vi "niWLAN - 80211abgnIQMeasurementsReadWrite.vi"(0 "niwlan analysis session":T3, 1 "file path (dialog if empty)":path, 2 "Measurement Type":T1(ring), 3 "PL":dbl, 7 "TV Parameters(DataType)":T2 {"Tx_Chan" format="%.0x"; "Standard" items=["80211A/G/J/P OFDM", "80211B/G DSSS", "80211G DSSSOFDM", "80211N MIMOOFDM", "80211AC MIMOOFDM"]; "OFDM Data Rate (Mbps)" items=["6", "9", "12", "18", "24", "36", "48", "54"]; "80211n PLCP Frame Format" items=["Mixed Format", "Greenfield Format"]; "FEC Coding Type" items=["BCC", "LDPC"]; "DSSS Data Rate (Mbps)" items=["1", "2", "5.5 CCK", "5.5 PBCC", "11 CCK", "11 PBCC", "22", "33"]}, 11 "error out":errorcluster, 12 "Measurement Time":dbl[](array[numeric]), 13 "First Row":bool=TRUE) -> (4 "niWLAN session":T3, 15 "error out":errorcluster)   [LabVIEW 2011]
uses:
  <vilib>/RF Toolkits/WLAN/analysis/controls/wlanv1 Analysis Refnum.ctl
  TV/RW/Includes/WLAN - TV - RW - INC - TV_DataType_Cluster.ctl
  <vilib>/Utility/file.llb/Write To Spreadsheet File (string).vi
  Program Files/National Instruments/LabVIEW 2011/resource/objmgr/niWLANAnalysis.rc
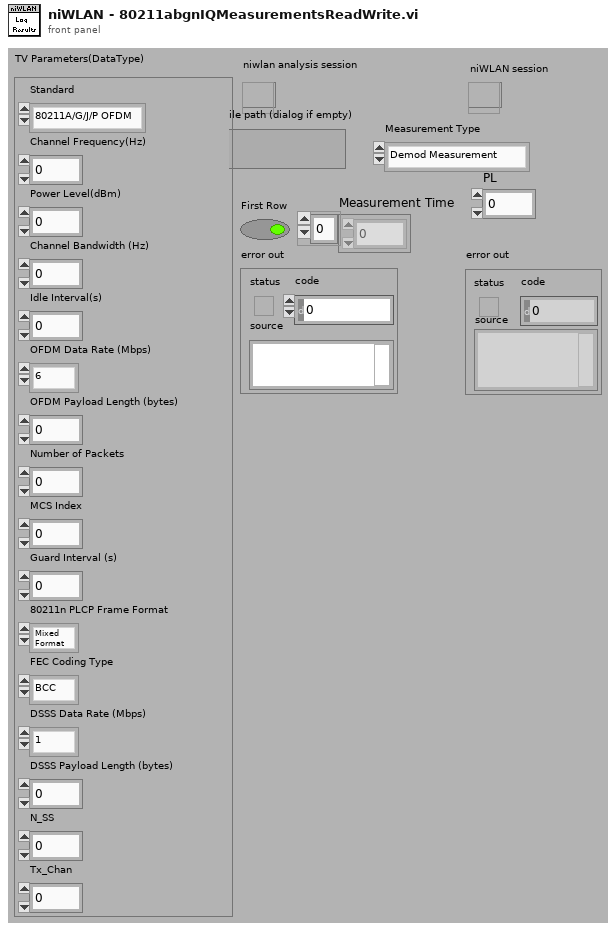
[diagram p1: front panel]
types:
  T1 = enum16{"Demod Measurement", "Spectrum Measurement"}
  T2 = typedef "WLAN - TV - RW - INC - TV_DataType_Cluster.ctl" = cluster{"Standard":i32, "Channel Frequency(Hz)":dbl, "Power Level(dBm)":dbl, "Channel Bandwidth (Hz)":dbl, "Idle Interval(s)":dbl, "OFDM Data Rate (Mbps)":i32, "OFDM Payload Length (bytes)":i32, "Number of Packets":i32, "MCS Index":i32, "Guard Interval (s)":dbl, "80211n PLCP Frame Format":i32, "FEC Coding Type":i32, "DSSS Data Rate (Mbps)":i32, "DSSS Payload Length (bytes)":i32, "N_SS":i32, "Tx_Chan":u32}
  T3 = typedef "wlanv1 Analysis Refnum.ctl" = refnum<k20>
  T4 = cluster{"subcarrier indices":i32[], "relative power (dB)":dbl[]}
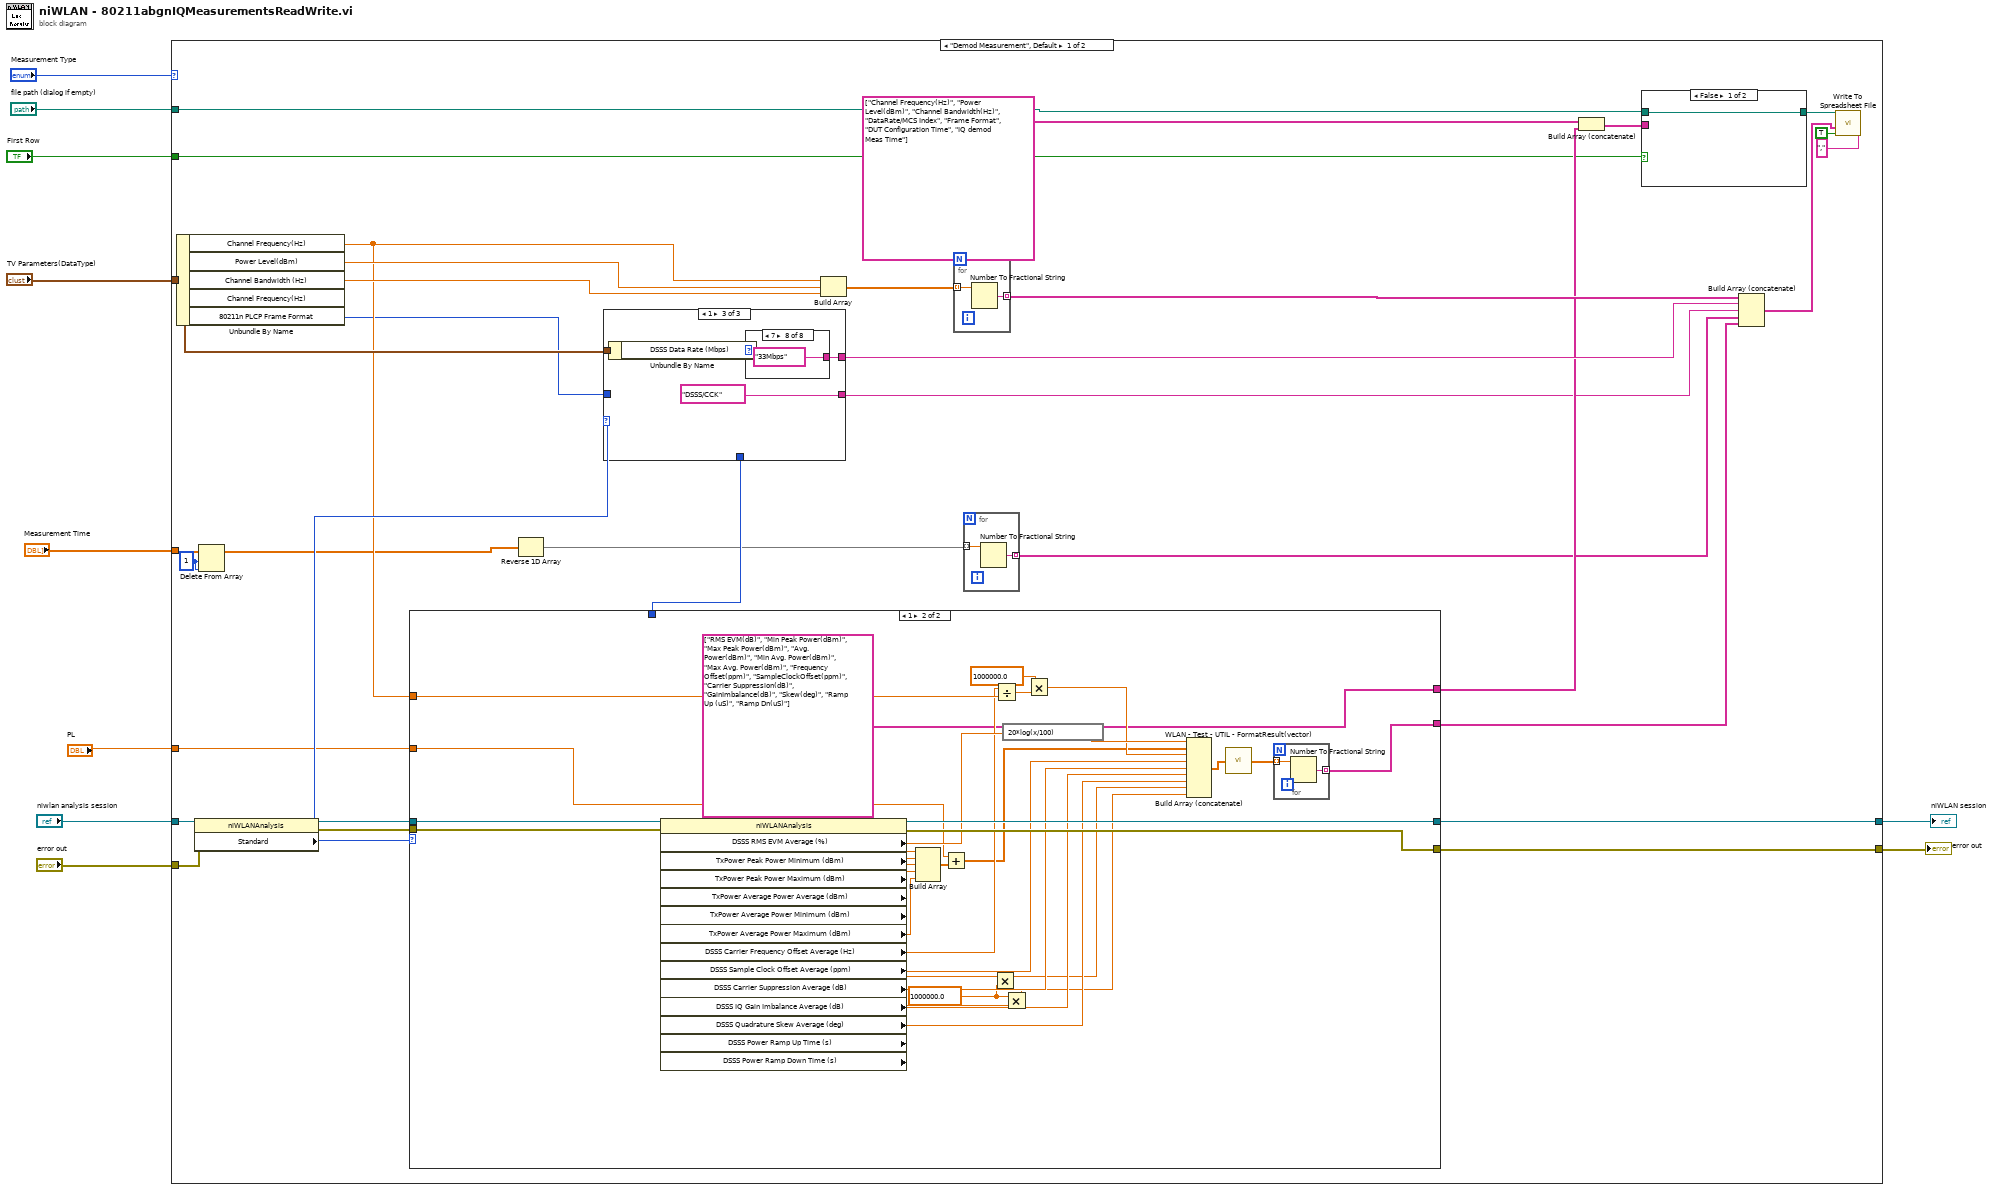
[diagram p0: block diagram]
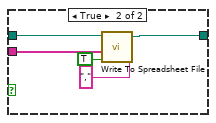
[diagram p2: hidden frame]
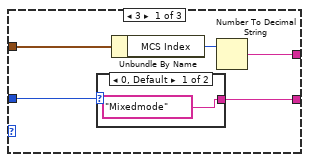
[diagram p3: hidden frame]
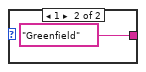
[diagram p4: hidden frame]
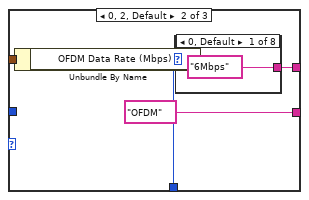
[diagram p5: hidden frame]
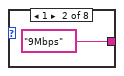
[diagram p6: hidden frame]
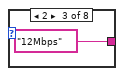
[diagram p7: hidden frame]
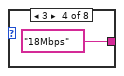
[diagram p8: hidden frame]
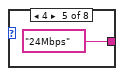
[diagram p9: hidden frame]
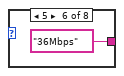
[diagram p10: hidden frame]
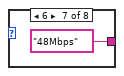
[diagram p11: hidden frame]
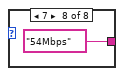
[diagram p12: hidden frame]
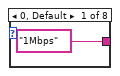
[diagram p13: hidden frame]
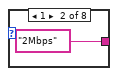
[diagram p14: hidden frame]
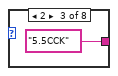
[diagram p15: hidden frame]
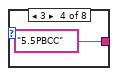
[diagram p16: hidden frame]
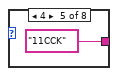
[diagram p17: hidden frame]
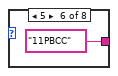
[diagram p18: hidden frame]
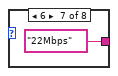
[diagram p19: hidden frame]
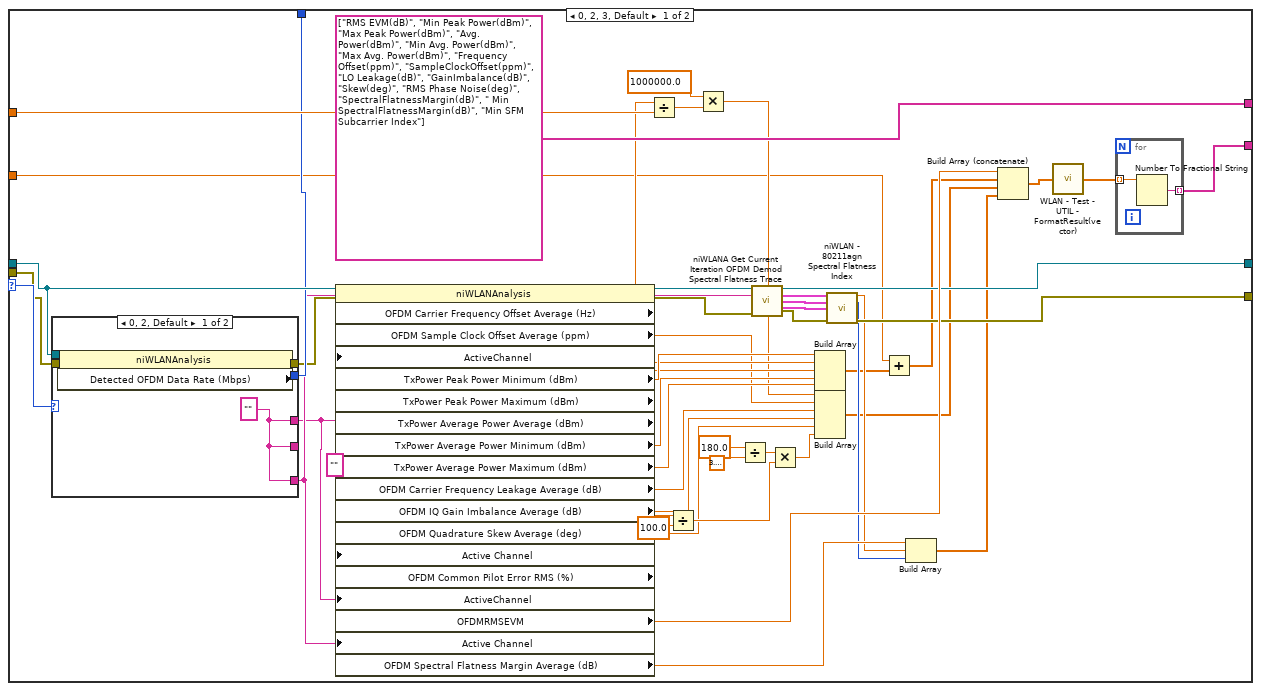
[diagram p20: hidden frame]
diagram:
  n1 = case shown="\"Demod Measurement\", Default" "Measurement Type" {
    tunnel: "niwlan analysis session" -> [w43 w226]
    tunnel: "error out" -> [w41 w227]
    tunnel: "TV Parameters(DataType)" -> [w34 w228]
    tunnel: [w28 w224] -> w7
    tunnel: [w27 w225] -> w6
    tunnel: "file path (dialog if empty)" -> [w21 w230]
    tunnel: "First Row" -> [w20 w229]
    tunnel: "Measurement Time" -> [w15 w186]
    tunnel: "PL" -> [w11 _]
    frame "Demod Measurement", Default {
      w14 = 1 ("length")
      n2 = Unbundle By Name(w34) -> ("Channel Frequency(Hz)"=w29:dbl, "Power Level(dBm)"=w38:dbl, "Channel Bandwidth (Hz)"=w37:dbl, "80211n PLCP Frame Format"=w18:i32)  [unwired: 1 out]
      n3 = property class="niWLANAnalysis"(reference=w43, error in=w41) -> (reference out=w42:T3, error out=w40:errorcluster, "Standard"=w33:i32)
      n4 = Delete From Array(array=w15, length=w14, index=w14) -> (array with subset deleted=w13:dbl[])  [unwired: 1 out]
      n5 = case shown="1" w33 {
        selector: w33 -> [w134 _]
        tunnel: w40 -> [w109 w176]
        tunnel: w42 -> [w111 w177]
        tunnel: [w106 w175] -> w28
        tunnel: [w102 w174] -> w27
        tunnel: [w132 w169] -> w32
        tunnel: [string[] ["RMS EVM(dB)", "Min Peak Power(dBm)", "Max Peak Power(dBm)", "Avg. Power(dBm)", "Min Avg. Power(dBm)", "Max Avg. Power(dBm)", "Frequency Offset(ppm)", "SampleClockOffset(ppm)", "LO Leakage(dB)", "GainImbalance(dB)", "Skew(deg)", "RMS Phase Noise(deg)", "SpectralFlatnessMargin(dB)", " Min SpectralFlatnessMargin(dB)", "Min SFM Subcarrier Index"] string[] ["RMS EVM(dB)", "Min Peak Power(dBm)", "Max Peak Power(dBm)", "Avg. Power(dBm)", "Min Avg. Power(dBm)", "Max Avg. Power(dBm)", "Frequency Offset(ppm)", "SampleClockOffset(ppm)", "Carrier Suppression(dB)", "GainImbalance(dB)", "Skew(deg)", "Ramp Up (uS)", "Ramp Dn(uS)"]] -> w30
        tunnel: w29 -> [w128 w166]
        tunnel: [w110 _] -> w19
        tunnel: w11 -> [w90 w151]
        frame 0, 2, 3, Default {
          n6 = case shown="0, 2, Default" w134 {
            tunnel: [w141 "Channel0/Stream0"] -> w104
            tunnel: [w141 "Stream0" ("Active Channel")] -> _
            tunnel: [w141 "Channel0" ("Active Channel")] -> w85
            tunnel: w111 -> [w140 _]
            tunnel: w109 -> [w139 w142]
            tunnel: [w138 _] -> w110
            tunnel: [w137 w142] -> w108
            frame 0, 2, Default {
              w141 = "" ("Active Channel")
              n7 = property class="niWLANAnalysis"(reference=w140, error in=w139) -> (error out=w137:errorcluster, "Detected OFDM Data Rate (Mbps)"=w138:i32)  [unwired: 1 out]
            }
            frame 3 {
            }
          }
          n8 = property class="niWLANAnalysis"(reference=w111, error in=w108, "ActiveChannel"=w85, "Active Channel"="", "ActiveChannel"=w85, "Active Channel"=w104) -> (reference out=w107:T3, error out=w105:errorcluster, "OFDM Carrier Frequency Offset Average (Hz)"=w113:dbl, "OFDM Sample Clock Offset Average (ppm)"=w95:dbl, "TxPower Peak Power Minimum (dBm)"=w125:dbl, "TxPower Peak Power Maximum (dBm)"=w124:dbl, "TxPower Average Power Average (dBm)"=w123:dbl, "TxPower Average Power Minimum (dBm)"=w122:dbl, "TxPower Average Power Maximum (dBm)"=w112:dbl, "OFDM Carrier Frequency Leakage Average (dB)"=w94:dbl, "OFDM IQ Gain Imbalance Average (dB)"=w93:dbl, "OFDM Quadrature Skew Average (deg)"=w92:dbl, "OFDM Common Pilot Error RMS (%)"=w114:dbl, "OFDMRMSEVM"=w133:dbl, "OFDM Spectral Flatness Margin Average (dB)"=w121:dbl)
          n9 = Divide(x=w113, y=w128) -> (x/y=w130:dbl)
          n10 = Divide(x=w114, y=100.0 ("x")) -> (x/y=w119:dbl)
          n11 = Multiply(x=1000000.0, y=w130) -> (x*y=w96:dbl)
          n12 = Divide(x=180.0, y=3.141592653589793) -> (x/y=w116:dbl)
          n13 = call <vilib>:"niWLANA Get Current Iteration OFDM Demod Spectral Flatness Trace.vi"("niwlan analysis session"=w107, "active channel"=w104, "error in"=w105) -> ("niwlan analysis session out"=w106:T3, "spectral flatness upper mask"=w101:T4, "spectral flatness trace"=w100:T4, "spectral flatness lower mask"=w99:T4, "error out"=w103:errorcluster)  [unwired: 8 in]
          n14 = Multiply(x=w116, y=w119) -> (x*y=w91:dbl)
          n15 = Build Array(w125, w124, w123, w122, w112) -> (w89:dbl[])
          n16 = Build Array(w96, w95, w94, w93, w92, w91) -> (w86:dbl[])
          n17 = call "niWLAN - 80211agn Spectral Flatness Index.vi"("spectral flatness upper mask"=w101, "spectral flatness Trace"=w100, "spectral flatness Lower mask"=w99, "error in (no error)"=w103) -> ("Least Spectral Flatness Margin"=w97:dbl, "Spectral Flatness Margin Subcarrier Index"=w98:i32, "error out"=w102:errorcluster)  [unwired: 9 in]
          n18 = Add(x=w90, y=w89) -> (x+y=w88:dbl[])
          n19 = Build Array(w121, w97, w98) -> (w87:dbl[])
          n20 = Build Array (concatenate)(w133, w88, w86, w87) -> (w127:dbl[])
          n21 = call "WLAN - Test - UTIL - FormatResult(vector).vi"("Number"=w127) -> ("2nd order decimal"=w126:dbl[])  [unwired: 14 in]
          n22 = for {
            tunnel: [w136] -> w132 mode=indexing
            tunnel: w126 -> [w135] mode=indexing
            n23 = Number To Fractional String(number=w135) -> (F-format string=w136:string)  [unwired: 3 in]
          }
        }
        frame 1 {
          w146 = 1000000.0 ("x")
          n24 = property class="niWLANAnalysis"(reference=w177, error in=w176) -> (reference out=w175:T3, error out=w174:errorcluster, "DSSS RMS EVM Average (%)"=w168:dbl, "TxPower Peak Power Minimum (dBm)"=w158:dbl, "TxPower Peak Power Maximum (dBm)"=w157:dbl, "TxPower Average Power Average (dBm)"=w156:dbl, "TxPower Average Power Minimum (dBm)"=w155:dbl, "TxPower Average Power Maximum (dBm)"=w154:dbl, "DSSS Carrier Frequency Offset Average (Hz)"=w163:dbl, "DSSS Sample Clock Offset Average (ppm)"=w173:dbl, "DSSS Carrier Suppression Average (dB)"=w172:dbl, "DSSS IQ Gain Imbalance Average (dB)"=w171:dbl, "DSSS Quadrature Skew Average (deg)"=w170:dbl, "DSSS Power Ramp Up Time (s)"=w150:dbl, "DSSS Power Ramp Down Time (s)"=w149:dbl)
          n25 = Build Array(w158, w157, w156, w155, w154) -> (w153:dbl[])
          n26 = Add(x=w151, y=w153) -> (x+y=w152:dbl[])
          n27 = Multiply(x=w150, y=w146) -> (x*y=w148:dbl)
          n28 = Divide(x=w163, y=w166) -> (x/y=w165:dbl)
          n29 = expression code="20*log(x/100)"(w168) -> (w167:dbl)
          n30 = Multiply(x=w146, y=w149) -> (x*y=w147:dbl)
          n31 = Multiply(x=1000000.0, y=w165) -> (x*y=w162:dbl)
          n32 = Build Array (concatenate)(w167, w152, w162, w173, w172, w171, w170, w148, w147) -> (w160:dbl[])
          n33 = call "WLAN - Test - UTIL - FormatResult(vector).vi"("Number"=w160) -> ("2nd order decimal"=w159:dbl[])  [unwired: 14 in]
          n34 = for {
            tunnel: [w179] -> w169 mode=indexing
            tunnel: w159 -> [w178] mode=indexing
            n35 = Number To Fractional String(number=w178) -> (F-format string=w179:string)  [unwired: 3 in]
          }
        }
      }
      n36 = Reverse 1D Array(array=w13) -> (reversed array=w12:dbl[])
      n37 = case shown="1" w33 {
        tunnel: [w56 "OFDM" ("active channel") "DSSS/CCK" ("active channel")] -> w17
        tunnel: w34 -> [w55 w61 w73]
        tunnel: [w53 w60 w71] -> w35
        tunnel: w19 -> [_ w59 _]
        tunnel: w18 -> [w52 _ _]
        frame 3 {
          n38 = case shown="0, Default" w52 {
            tunnel: ["Mixedmode" ("active channel") "Greenfield" ("active channel")] -> w56
            frame 0, Default {
            }
            frame 1 {
            }
          }
          n39 = Unbundle By Name(w55) -> ("MCS Index"=w54:i32)
          n40 = Number To Decimal String(number=w54) -> (decimal integer string=w53:string)  [unwired: 1 in]
        }
        frame 0, 2, Default {
          n41 = Unbundle By Name(w61) -> ()  [unwired: 1 out]
          n42 = case shown="0, Default" w59 {
            tunnel: ["6Mbps" ("active channel") "9Mbps" ("active channel") "12Mbps" ("active channel") "18Mbps" ("active channel") "24Mbps" ("active channel") "36Mbps" ("active channel") "48Mbps" ("active channel") "54Mbps" ("active channel")] -> w60
            frame 0, Default {
            }
            frame 1 {
            }
            frame 2 {
            }
            frame 3 {
            }
            frame 4 {
            }
            frame 5 {
            }
            frame 6 {
            }
            frame 7 {
            }
          }
        }
        frame 1 {
          n43 = Unbundle By Name(w73) -> ("DSSS Data Rate (Mbps)"=w72:i32)
          n44 = case shown="7" w72 {
            tunnel: ["1Mbps" ("active channel") "2Mbps" ("active channel") "5.5CCK" ("active channel") "5.5PBCC" ("active channel") "11CCK" ("active channel") "11PBCC" ("active channel") "22Mbps" ("active channel") "33Mbps" ("active channel")] -> w71
            frame 0, Default {
            }
            frame 1 {
            }
            frame 2 {
            }
            frame 3 {
            }
            frame 4 {
            }
            frame 5 {
            }
            frame 6 {
            }
            frame 7 {
            }
          }
        }
      }
      n45 = Build Array(w29, w38, w37) -> (w39:dbl[])
      n46 = for {
        tunnel: [w84] -> w36 mode=indexing
        tunnel: w39 -> [w83] mode=indexing
        n47 = Number To Fractional String(number=w83) -> (F-format string=w84:string)  [unwired: 3 in]
      }
      n48 = for {
        tunnel: [w45] -> w16 mode=indexing
        tunnel: w12 -> [w44] mode=indexing
        n49 = Number To Fractional String(number=w44) -> (F-format string=w45:string)  [unwired: 3 in]
      }
      n50 = Build Array (concatenate)(string[] ["Channel Frequency(Hz)", "Power Level(dBm)", "Channel Bandwidth(Hz)", "DataRate/MCS Index", "Frame Format", "DUT Configuration Time", "IQ demod Meas Time"], w30) -> (w26:string[])
      n51 = case shown="False" w20 {
        tunnel: w21 -> [w46 w49]
        tunnel: [w46 w50] -> w23
        tunnel: w26 -> [_ w47]
        frame False {
        }
        frame True {
          n52 = call-poly <vilib>:"Write To Spreadsheet File.vi"("delimiter (\\t)"="," ("delimiter (\\t)"), "append to file? (new file:F)"=TRUE, "1D data"=w47, "file path (dialog if empty)"=w49) -> ("new file path (Not A Path if cancelled)"=w50:path)  [unwired: 4 in]
        }
      }
      n53 = Build Array (concatenate)(w36, w35, w17, w16, w32) -> (w22:string[])
      n54 = call-poly <vilib>:"Write To Spreadsheet File.vi"("delimiter (\\t)"="," ("delimiter (\\t)"), "append to file? (new file:F)"=TRUE, "1D data"=w22, "file path (dialog if empty)"=w23) -> ()  [unwired: 4 in, 1 out]
    }
    frame "Spectrum Measurement" {
      n55 = property class="niWLANAnalysis"(reference=w226, error in=w227) -> (reference out=w223:T3, error out=w222:errorcluster, "Standard"=w221:i32)
      n56 = Array Subset(array=w186, index=1) -> (w184:dbl[])  [unwired: 1 in]
      n57 = Reverse 1D Array(array=w184) -> (reversed array=w180:dbl[])
      n58 = for {
        tunnel: [w232] -> w182 mode=indexing
        tunnel: w180 -> [w231] mode=indexing
        n59 = Number To Fractional String(number=w231) -> (F-format string=w232:string)  [unwired: 3 in]
      }
      n60 = case shown="0, 2, Default" w221 {
        tunnel: ["Channel0" ("active channel") "" ("active channel") "" ("active channel")] -> w192
        tunnel: w228 -> [w250 w258 w272]
        tunnel: [w246 w256 w270] -> w196
        tunnel: [string[] ["SMM(dB)(-33MHz  -  -30MHz) ", "SMM(dB)(-30MHz  -  -20MHz) ", "SMM(dB)(-20MHz  -  -11MHz) ", "SMM(dB)(-11MHz  -  9MHz) ", "SMM(dB)(-9MHz  -  9MHz) ", "SMM(dB)(9MHz  -  11MHz) ", "SMM(dB)(11MHz  -  20MHz) ", "SMM(20MHz  -  33MHz) "] string[] ["SMM(dB)(-33MHz  -  -30MHz) ", "SMM(dB)(-30MHz  -  -20MHz) ", "SMM(dB)(-20MHz  -  -11MHz) ", "SMM(dB)(-11MHz  -  9MHz) ", "SMM(dB)(-9MHz  -  9MHz) ", "SMM(dB)(9MHz  -  11MHz) ", "SMM(dB)(11MHz  -  20MHz) ", "SMM(20MHz  -  30Hz) ", "SMM(30MHz  -  33MHz) "] string[] ["SMM(-33MHz  -  -22MHz) ", "SMM(-22MHz  -  -11MHz) ", "SMM(-11MHz  -  11MHz) ", "SMM(11MHz  -  22MHz) ", "SMM(22MHz  -  33MHz) "]] -> w191
        tunnel: [w244 "OFDM" ("active channel") "DSSS/CCK" ("active channel")] -> w183
        frame 3 {
          n61 = Unbundle By Name(w250) -> ("MCS Index"=w249:i32, "80211n PLCP Frame Format"=w245:i32)
          n62 = case shown="0, Default" w245 {
            tunnel: ["Mixedmode" ("active channel") "Greenfield" ("active channel")] -> w244
            frame 0, Default {
            }
            frame 1 {
            }
          }
          n63 = Number To Decimal String(number=w249) -> (decimal integer string=w247:string)  [unwired: 1 in]
          n64 = Concatenate Strings("MCS " ("string"), w247) -> (w246:string)
        }
        frame 0, 2, Default {
          n65 = Unbundle By Name(w258) -> ("OFDM Data Rate (Mbps)"=w257:i32)
          n66 = case shown="7" w257 {
            tunnel: ["6Mbps" ("active channel") "9Mbps" ("active channel") "12Mbps" ("active channel") "18Mbps" ("active channel") "24Mbps" ("active channel") "36Mbps" ("active channel") "48Mbps" ("active channel") "54Mbps" ("active channel")] -> w256
            frame 0, Default {
            }
            frame 1 {
            }
            frame 2 {
            }
            frame 3 {
            }
            frame 4 {
            }
            frame 5 {
            }
            frame 6 {
            }
            frame 7 {
            }
          }
        }
        frame 1 {
          n67 = Unbundle By Name(w272) -> ("DSSS Data Rate (Mbps)"=w271:i32)
          n68 = case shown="7" w271 {
            tunnel: ["1Mbps" ("active channel") "2Mbps" ("active channel") "5.5CCK" ("active channel") "5.5PBCC" ("active channel") "11CCK" ("active channel") "11PBCC" ("active channel") "22Mbps" ("active channel") "33Mbps" ("active channel")] -> w270
            frame 0, Default {
            }
            frame 1 {
            }
            frame 2 {
            }
            frame 3 {
            }
            frame 4 {
            }
            frame 5 {
            }
            frame 6 {
            }
            frame 7 {
            }
          }
        }
      }
      n69 = property class="niWLANAnalysis"(reference=w223, error in=w222, "Active Channel"=w192) -> (reference out=w219:T3, error out=w220:errorcluster, "Spectral Mask Margin (dB)"=w188:dbl, "Spectral Mask Margin Vector"=w187:dbl[])
      n70 = call <vilib>:"niWLANA Get Spectral Mask Trace.vi"("niwlan analysis session"=w219, "active channel"=w192, "error in"=w220) -> ("niwlan analysis session out"=w224:T3, "spectral mask"=w218:cluster{"f0":dbl, "df":dbl, "Y":dbl[]}[], "error out"=w225:errorcluster)  [unwired: 10 in]
      n71 = Index Array(array=w218) -> (element #1=w217:cluster{"f0":dbl, "df":dbl, "Y":dbl[]}, element #2=w216:cluster{"f0":dbl, "df":dbl, "Y":dbl[]})  [unwired: 2 in]
      n72 = Build Array (concatenate)(string[] ["Channel Frequency(Hz)", "Power Level(dBm)", "Channel BW(Hz)", "DataRate/MCS Index", "Frame Format", "DUT Configuration Time", "IQ Spectrum Meas Time", "SM Violation(%) ", "SMM(dB)"], w191) -> (w193:string[])
      n73 = case shown="True" w229 {
        tunnel: w230 -> [w233 w237]
        tunnel: [w233 w238] -> w195
        tunnel: w193 -> [_ w234]
        frame False {
        }
        frame True {
          n74 = call-poly <vilib>:"Write To Spreadsheet File.vi"("delimiter (\\t)"="," ("delimiter (\\t)"), "append to file? (new file:F)"=TRUE, "1D data"=w234, "file path (dialog if empty)"=w237) -> ("new file path (Not A Path if cancelled)"=w238:path)  [unwired: 4 in]
        }
      }
      n75 = Build Array (concatenate)(w183, w182) -> (w181:string[])
      n76 = Unbundle By Name(w217) -> ("Y"=w215:dbl[])
      n77 = Unbundle By Name(w216) -> ("Y"=w210:dbl[])
      n78 = Subtract(x=w215, y=w210) -> (x-y=w214:dbl[])
      n79 = Array Size(array=w210) -> (size(s)=w209:i32)
      n80 = Less Than 0?(x=w214) -> (x < 0?=w213:bool[])
      n81 = Boolean To (0,1)(Boolean=w213) -> (0, 1=w212:i16[])
      n82 = Add Array Elements(numeric array=w212) -> (sum=w211:i16)
      n83 = Unbundle By Name(w228) -> ("Channel Frequency(Hz)"=w202:dbl, "Power Level(dBm)"=w201:dbl, "Channel Bandwidth (Hz)"=w200:dbl)
      n84 = Divide(x=w211, y=w209) -> (x/y=w208:dbl)
      n85 = Multiply(x=w208, y=100.0) -> (x*y=w206:dbl)
      n86 = Build Array (concatenate)(w206, w188, w187) -> (w190:dbl[])
      n87 = call "WLAN - Test - UTIL - FormatResult(vector).vi"("Number"=w190) -> ("2nd order decimal"=w189:dbl[])  [unwired: 14 in]
      n88 = Build Array(w202, w201, w200) -> (w203:dbl[])
      n89 = for {
        tunnel: [w240] -> w199 mode=indexing
        tunnel: w203 -> [w239] mode=indexing
        n90 = Number To Fractional String(number=w239) -> (F-format string=w240:string)  [unwired: 3 in]
      }
      n91 = for {
        tunnel: [w242] -> w197 mode=indexing
        tunnel: w189 -> [w241] mode=indexing
        n92 = Number To Fractional String(number=w241) -> (F-format string=w242:string)  [unwired: 3 in]
      }
      n93 = Build Array (concatenate)(w199, w196, w181, w197) -> (w198:string[])
      n94 = call-poly <vilib>:"Write To Spreadsheet File.vi"("delimiter (\\t)"="," ("delimiter (\\t)"), "append to file? (new file:F)"=TRUE, "1D data"=w198, "file path (dialog if empty)"=w195) -> ()  [unwired: 4 in, 1 out]
    }
  }
  "error out" <- w6
  "niWLAN session" <- w7
